vi "Request Response.vi"() -> ()   [LabVIEW 2024]
uses:
  Controls/nats message.ctl
  Controls/msg type.ctl
  NATS Subscription/NATS Subscription.lvclass
  NATS Subscription/NATS Subscription.lvclass/NATS Subscription.ctl
  NATS Subscription/get id.vi
  NATS Client/NATS Client.lvclass
  NATS Core.lvlib
panel:
  out "subscription response":T1
  in  "reply subject":string="wham.whoop"
  out "nats message":T1
  in  "request subject":string
  in  "payload":string
  in  "request":bool
  in  "unsub":bool
  in  "subject":string
  in  "sub":bool
  out "error out":errorcluster
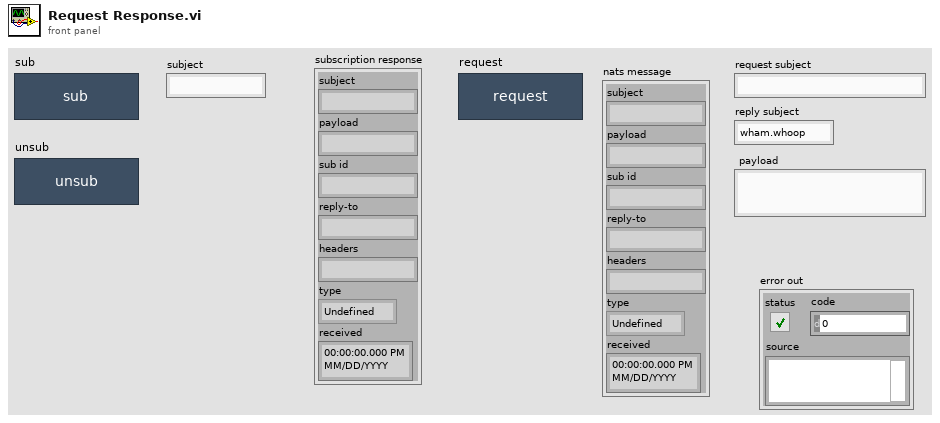
[diagram p1: front panel]
types:
  T1 = typedef "NATS Core.lvlib/nats message.ctl" = cluster{"subject":string, "payload":string, "sub id":string, "reply-to":string, "headers":string, "type":T2, "received":timestamp}
  T2 = typedef "NATS Core.lvlib/msg type.ctl" = enum16{"Undefined", "MSG", "HMSG", "+OK", "PING", "PONG", "-ERR", "INFO"}
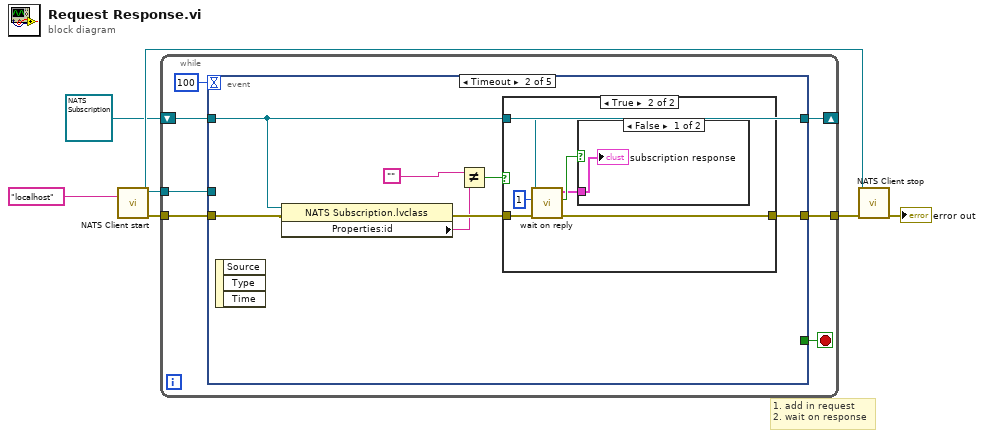
[diagram p0: block diagram]
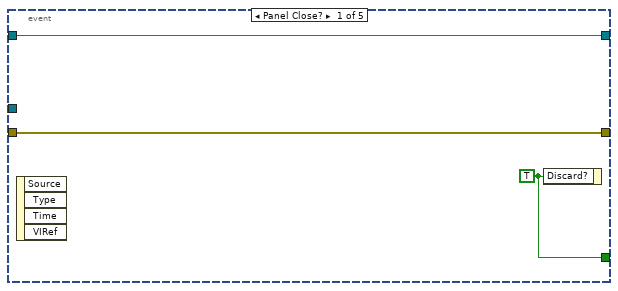
[diagram p2: hidden frame]
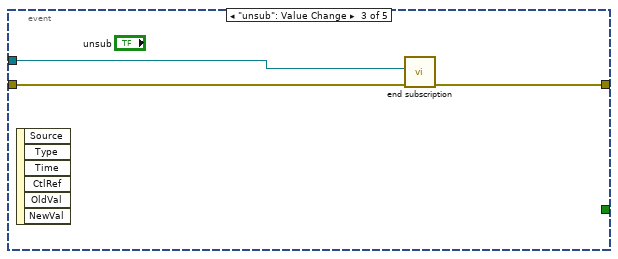
[diagram p5: hidden frame]
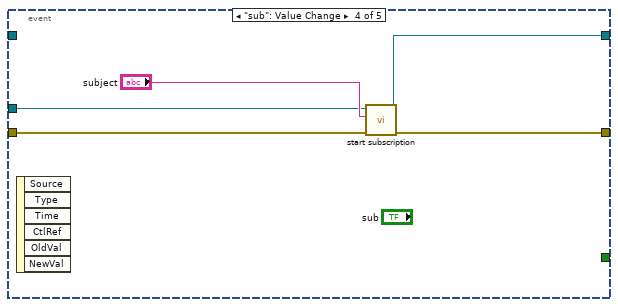
[diagram p6: hidden frame]
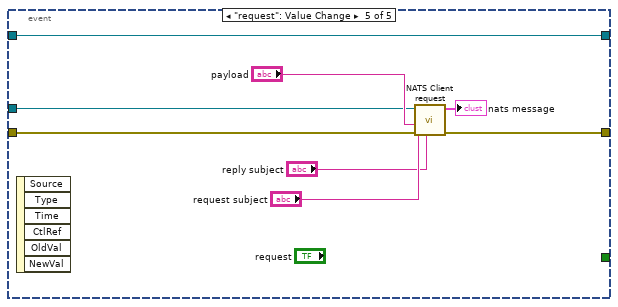
[diagram p7: hidden frame]
diagram:
  # "1. add in request\n2. wait on response"
  n1 = call "NATS Client start.vi"("address"="localhost") -> ("error out"=w6:errorcluster, "NATS Client out"=w2:refnum<class "NATS Client.lvclass">)  [unwired: 9 in]
  n2 = while {
    tunnel: w6 -> [w12]
    tunnel: [w11] -> w3
    tunnel: w2 -> [w10]
    shift-right: [w8] -> _
    shift-left: refnum<class "NATS Subscription.lvclass"> refnum ("NATS Subscription") -> [w7]
    stop <- w13 stop-if-true
    n3 = event shown="[1] Timeout" {
      selector: _ -> [_ _ _ _ _]
      dyn-events: _ -> [_ _ _ _ _]
      timeout: 100 -> [_ _ _ _ _]
      tunnel: [w16 _ _ _ _] -> w13
      tunnel: [w15 w23 w33 w38 w46] -> w11
      tunnel: w12 -> [w15 w20 w32 w39 w47]
      tunnel: w10 -> [_ _ w34 w36 w42]
      tunnel: [w14 w22 _ w35 w40] -> w8
      tunnel: w7 -> [w14 w22 _ _ w40]
      event Panel Close? {
        w16 = TRUE ("Discard?")
        n4 = event-data() -> ()  [unwired: 1 in, 4 out]
        n5 = event-data("Discard?"=w16) -> ()  [unwired: 1 in, 1 out]
      }
      event Timeout {
        n6 = event-data() -> ()  [unwired: 1 in, 3 out]
        n7 = property class="NATS Subscription.lvclass"(reference=w22, error in=w20) -> (error out=w21:errorcluster, "Properties:id"=w19:string)  [unwired: 1 out]
        n8 = Not Equal?(x="", y=w19) -> (x != y?=w17:bool)
        n9 = case shown="True" w17 {
          tunnel: [w24 w30] -> w23
          tunnel: w22 -> [_ w29]
          tunnel: w21 -> [w24 w28]
          frame False {
          }
          frame True {
            n10 = call-dynamic "wait on reply.vi"("error in"=w28, "timeout in ms (-1)"=1, "NATS Subscriber in"=w29) -> ("error out"=w30:errorcluster, "time out"=w26:bool, "nats message"=w25:T1)  [unwired: 6 in]
            n11 = case shown="False" w26 {
              tunnel: w25 -> [w31 _]
              frame False {
                "subscription response" <- w31
              }
              frame True {
              }
            }
          }
        }
      }
      event "unsub": Value Change {
        n12 = event-data() -> ()  [unwired: 1 in, 6 out]
        n13 = call "end subscription.vi"("error in"=w32, "NATS Client"=w34) -> ("error out"=w33:errorcluster)  [unwired: 9 in]
      }
      event "sub": Value Change {
        n14 = event-data() -> ()  [unwired: 1 in, 6 out]
        n15 = call "start subscription.vi"("error in"=w39, "subject"="subject", "NATS Client"=w36) -> ("error out"=w38:errorcluster, "NATS Subscription"=w35:refnum<class "NATS Subscription.lvclass">)  [unwired: 7 in]
      }
      event "request": Value Change {
        n16 = event-data() -> ()  [unwired: 1 in, 6 out]
        n17 = call "NATS Client request.vi"("reply subject"="reply subject", "error in"=w47, "payload"="payload", "subject"="request subject", "NATS Client in"=w42) -> ("error out"=w46:errorcluster, "nats message"=→"nats message":T1)  [unwired: 4 in, 1 out]
      }
    }
  }
  n18 = call "NATS Client stop.vi"("error in"=w3, "NATS Client"=w2) -> ("error out"=→"error out":errorcluster)  [unwired: 9 in]
